vi "RealSense_HelloWorld_Left_Right_unrectified.vi"() -> ()   [LabVIEW 2017]
doc: "This demo shows how to connect a RealSense D4xx Stereo Depth Camera, and stream the LEFT and the RIGHT raw unrectified images."
uses:
  <vilib>/picture/picture.llb/Draw True-Color Pixmap.vi
  libRealSense3.lvlib
panel:
  in  "autoexposure":bool
  in  "Gain (16-248)":sgl=16.0
  in  "Exposure,us":sgl=33000.0
  in  "Tab Control":enum32{"Monochrome L+R", "Intensity Chart L"}(tab)
  in  "Zoom Factor":sgl=0.29
  out "Unrect L":picture
  out "Unrect R":picture
  out "LEFT IMAGE":sgl[][](graph)
  out "RIGHT IMAGE":sgl[][](graph)
  out "iteration":i32=1
  in  "stop":bool=TRUE
  out "release frame error":string="No Error"
  out "Capture1 Error":string="No Error"
  out "Config error":string="No Error\rNo Error"
  out "init results":T1={"camera name"="Intel RealSense 415", "camera S/N"="725112060291", "F/W"="05.08.09.00", "Sensor name"="Stereo Module", "api_version"=20710, "rscontext"=657762304, "device_list"=395444960, "device count"=2, "Dev out"=657678208, "sensor_list"=657686400, "sensor count"=2, "Sensor out"=657915824}
  out "init error":string="No Error\rNo Error\rNo Error\rNo Error\rNo Error\rNo Error\rNo Error\rNo Error\rNo Error\rNo Error\rNo Error"
  out "Close Error":string="No Error\rNo Error\rNo Error\rNo Error"
  out "Start Error":string="No Error\rNo Error\rNo Error"
  out "Capture2 error":string="No Error"
  in  "Select Resolution":u16(ring)=3 items=["960 x 540 @15fps", "960 x 540 @25fps", "1920 x 1080 @15fps", "1920 x 1080 @25fps"]
  # "RealSense Hello World: Left-Right UnRectified"
  # "This demo shows how to connect a RealSense D4xx Stereo Depth Camera, and stream the LEFT and the RIGHT raw unrectified images. Zoom in and scroll the horizontal/vertical bar to look at different parts of image. The images are the input images to the stereo algorithm. They are not rectified by ASIC.  They can be used to look at raw image quality before any processing."
  # "Use this to ZOOM and move image"
  # "Use this to ZOOM and move image"
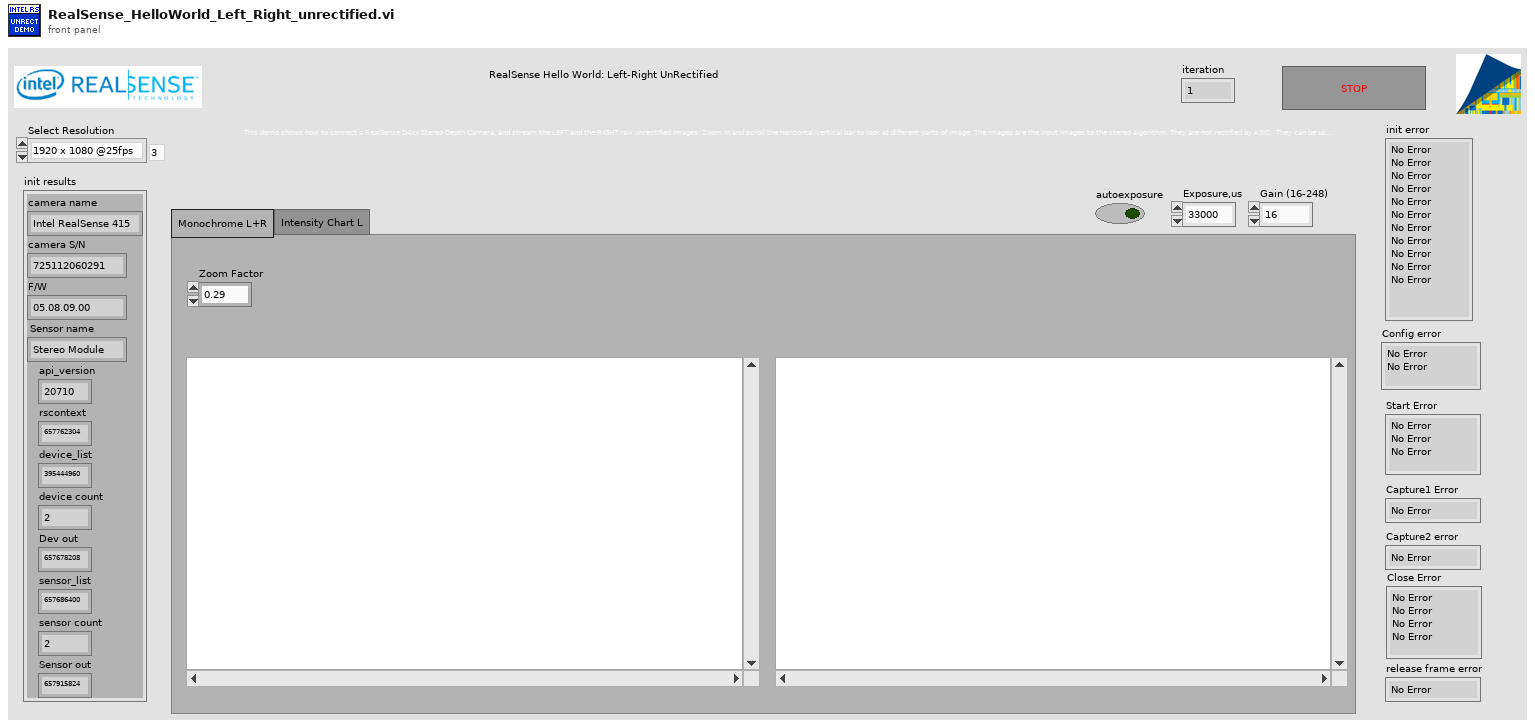
[diagram p1: front panel]
types:
  T1 = cluster{"camera name":string, "camera S/N":string, "F/W":string, "Sensor name":string, "api_version":i32, "rscontext":u64, "device_list":u64, "device count":i32, "Dev out":u64, "sensor_list":u64, "sensor count":i32, "Sensor out":u64}
  T2 = enum16{"Depth", "Color (ext.)", "Color (left) ", "IR Left", "IR Right", "IR Left (Y16)", "IR Right (Y16)"}
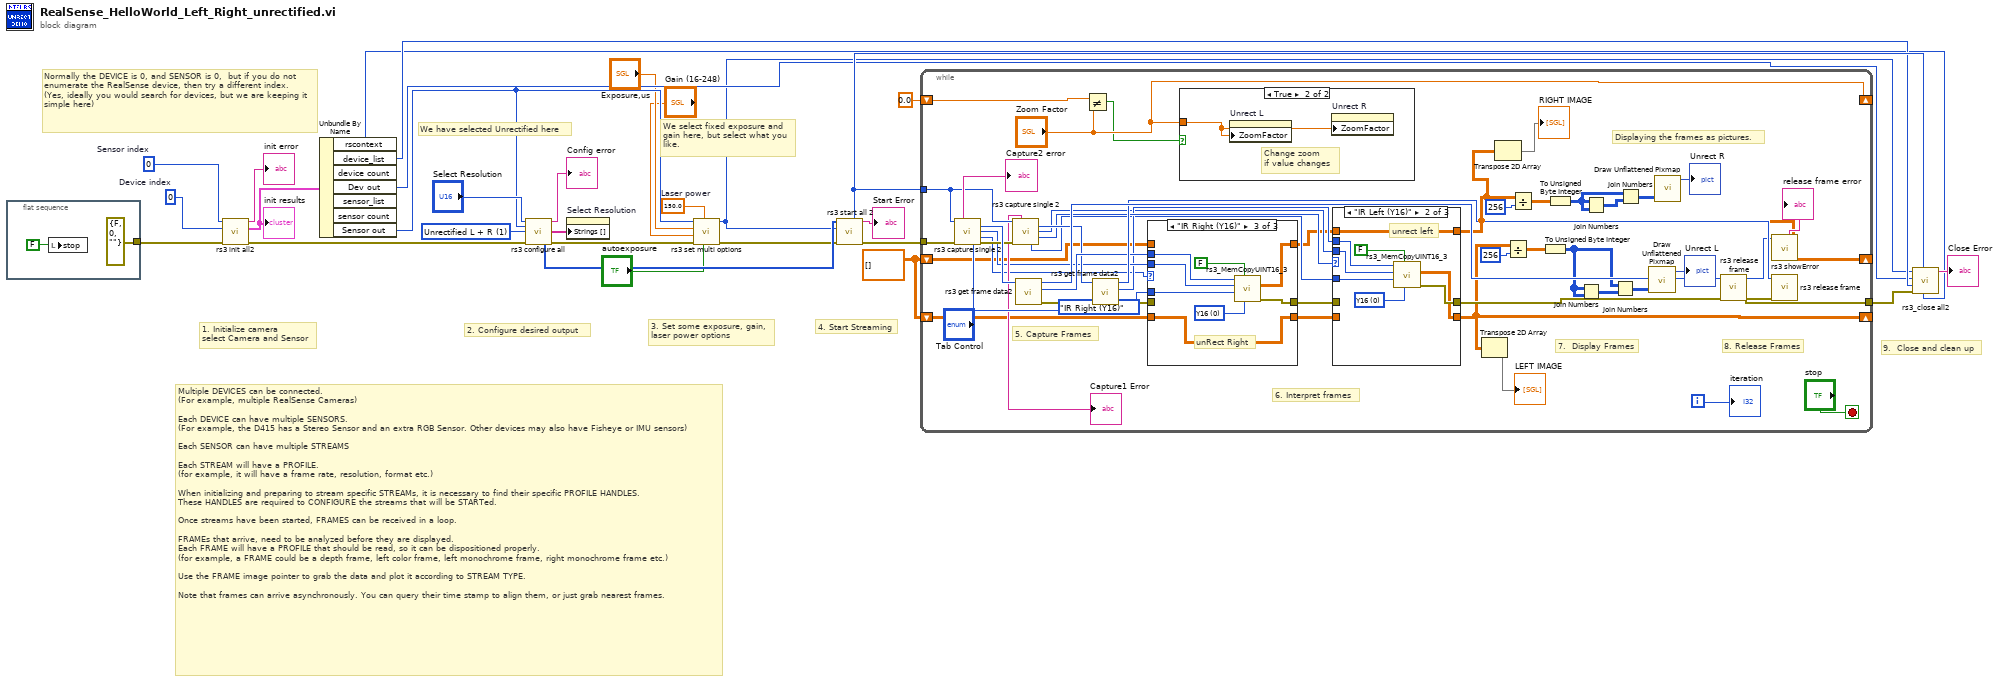
[diagram p0: block diagram]
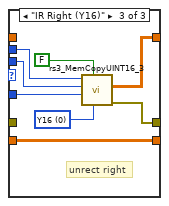
[diagram p4: hidden frame]
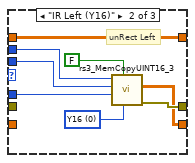
[diagram p6: hidden frame]
diagram:
  w29 = 0  # Device index
  w28 = 0  # Sensor index
  w4 = sgl 150.0  # Laser power
  w10 = u16 1 items=["Depth + Left Color", "Unrectified L + R", "Rectified L + R"] ("Stream selection")
  w11 = sgl[][] [] ("2D Array Output")
  # "We select fixed exposure and gain here, but select what you like."
  # "We have selected Unrectified here"
  # "Normally the DEVICE is 0, and SENSOR is 0,  but if you do not enumerate the RealSense device, then try a different index.\n(Yes, ideally you would search for devices, but we are keeping it simple here)"
  # "Multiple DEVICES can be connected. \n(For example, multiple RealSense Cameras)\n\nEach DEVICE can have multiple SENSORS. \n(For example, the D415 has a Stereo Sensor and an extra RGB Sensor. Other devices may also have Fisheye or IMU sensors) \n\nEach SENSOR can have multiple STREAMS\n\nEach STREAM will have a PROFILE. \n(for example, it will have a frame rate, resolution, format etc.)\n\nWhen initializing and preparing to stream specific STREAMs, it is necessary to find their specific PROFILE HANDLES.\nThese HANDLES are required to CONFIGURE the streams that will be STARTed. \n\nOnce streams have been started, FRAMES can be received in a loop. \n \nFRAMEs that arrive, need to be analyzed before they are displayed. \nEach FRAME will have a PROFILE that should be read, so it can be dispositioned properly.\n(for example, a FRAME could be a depth frame, left color frame, left monochrome frame, right monochrome frame etc.)\n\nUse the FRAME image pointer to grab the data and plot it according to STREAM TYPE.\n\nNote that frames can arrive asynchronously. You can query their time stamp to align them, or just grab nearest frames."
  # "9.  Close and clean up"
  # "4. Start Streaming"
  # "3. Set some exposure, gain, \nlaser power options"
  # "2. Configure desired output"
  # "1. Initialize camera\nselect Camera and Sensor"
  n1 = flat-sequence {
    tunnel: [errorcluster {"status"=FALSE, "code"=0, "source"=""} ("error in")] -> w12
    frame #0 {
      n2 = local write "stop"(FALSE ("stop")) -> ()
    }
  }
  n3 = call "rs3 init all2.vi"("error in"=w12, "Select Device"=w29, "Select Sensor"=w28) -> ("error out"=w27:errorcluster, "init results"=w20:T1, "init error"=→"init error":string)  [unwired: 2 in, 4 out]
  "init results" <- w20
  n4 = Unbundle By Name(w20) -> ("rscontext"=w18:u64, "device_list"=w19:u64, "Dev out"=w15:u64, "Sensor out"=w7:u64)  [unwired: 3 out]
  n5 = call "rs3 configure all.vi"("Select Resolution"="Select Resolution", "Sensor in"=w7, "Stream selection"=w10, "error in (no error)"=w27) -> ("config error"=→"Config error":string, "Output stream"=w13:string[], "Stream Profile Handles"=w26:u64[], "error out"=w9:errorcluster)  [unwired: 2 in, 6 out]
  n6 = property on="Select Resolution" class="Ring (strict)"("Strings []"=w13) -> ()  [unwired: 2 in, 2 out]
  n7 = call "rs3 set multi options.vi"("autoexposure"="autoexposure", "Laser power, mW (0-360)"=w4, "error in (no error)"=w9, "Gain(16-248)"="Gain (16-248)", "Exposure, us"="Exposure,us", "Sensor in"=w7) -> ("error out"=w8:errorcluster, "Sensor out"=w6:u64)  [unwired: 3 in, 1 out]
  n8 = call "rs3 start all 2.vi"("error in (no error)"=w8, "Sensor in"=w6, "Stream profile array"=w26) -> ("error out"=w14:errorcluster, "Config Error"=→"Start Error":string, "queue out"=w25:u64)  [unwired: 5 in, 1 out]
  n9 = while {
    tunnel: w25 -> [w68]
    tunnel: w14 -> [w81]
    tunnel: [w73] -> w24
    shift-right: [w33] -> _
    shift-left: w11 -> [w54]
    shift-right: [w35] -> _
    shift-left: w11 -> [w52]
    shift-right: ["Zoom Factor"] -> _
    shift-left: sgl 0.0 ("Zoom Factor") -> [w38]
    i -> [w79]
    stop <- "stop" stop-if-true
    (unwired) T2."IR Right (Y16)" ("Stream type")
    # "Displaying the frames as pictures."
    # "8. Release Frames"
    # "7.  Display Frames"
    # "6. Interpret frames"
    # "5. Capture Frames"
    n10 = call "rs3 capture single 2.vi"("queue in"=w68, "error in (no error)"=w81) -> ("Capture Error"=→"Capture2 error":string, "frame out"=w78:u64, "width"=w65:i32, "Stream type"=w55:T2, "height"=w75:i32, "error out"=w69:errorcluster)  [unwired: 2 in, 6 out]
    n11 = call "rs3 capture single 2.vi"("queue in"=w68, "error in (no error)"=w69) -> ("Capture Error"=→"Capture1 Error":string, "frame out"=w66:u64, "width"=w57:i32, "Stream type"=w59:T2, "height"=w56:i32)  [unwired: 2 in, 7 out]
    n12 = call "rs3 get frame data2.vi"("frame in"=w78) -> ("error out"=w72:errorcluster, "image pointer out"=w76:u64, "Frame out"=w80:u64)  [unwired: 7 in, 1 out]
    n13 = Not Equal?(x=w38, y="Zoom Factor") -> (x != y?=w36:bool)
    n14 = call "rs3 get frame data2.vi"("error in (no error)"=w72, "frame in"=w66) -> ("error out"=w71:errorcluster, "image pointer out"=w58:u64, "Frame out"=w77:u64)  [unwired: 6 in, 1 out]
    n15 = case shown="\"IR Right (Y16)\"" w55 {
      tunnel: [w104 w111 w119] -> w61
      tunnel: w76 -> [_ w110 w118]
      tunnel: w65 -> [_ w109 w117]
      tunnel: w75 -> [_ w108 w116]
      tunnel: w71 -> [w104 _ _]
      tunnel: [w103 w107 w114] -> w53
      tunnel: w54 -> [w103 _ w114]
      tunnel: w52 -> [w102 w106 _]
      tunnel: [w102 w106 w115] -> w51
      frame "Color (ext.)", Default {
      }
      frame "IR Left (Y16)" {
        w112 = u16 0 items=["Y16", "Y8"] ("Image format")
        # "unRect Left"
        n16 = call "rs3_MemCopyUINT16_3.vi"("Image format"=w112, "Transpose"=FALSE, "Depth Y"=w108, "Depth X"=w109, "Zimage pointer"=w110) -> ("error out"=w111:errorcluster, "2D Array Output"=w107:sgl[][])  [unwired: 3 in, 2 out]
      }
      frame "IR Right (Y16)" {
        w120 = u16 0 items=["Y16", "Y8"] ("Image format")
        # "unRect Right"
        n17 = call "rs3_MemCopyUINT16_3.vi"("Image format"=w120, "Transpose"=FALSE, "Depth Y"=w116, "Depth X"=w117, "Zimage pointer"=w118) -> ("error out"=w119:errorcluster, "2D Array Output"=w115:sgl[][])  [unwired: 3 in, 2 out]
      }
    }
    n18 = case shown="True" w36 {
      tunnel: "Zoom Factor" -> [_ w82]
      frame False {
      }
      frame True {
        # "Change zoom\nif value changes"
        n19 = property on="Unrect L" class="Pict"("ZoomFactor"=w82) -> ()  [unwired: 2 in, 2 out]
        n20 = property on="Unrect R" class="Pict"("ZoomFactor"=w82) -> ()  [unwired: 2 in, 2 out]
      }
    }
    n21 = case shown="\"IR Left (Y16)\"" w59 {
      tunnel: [w85 w92 w100] -> w60
      tunnel: w58 -> [_ w91 w99]
      tunnel: w57 -> [_ w90 w98]
      tunnel: w56 -> [_ w89 w97]
      tunnel: w61 -> [w85 _ _]
      tunnel: w53 -> [w84 _ w95]
      tunnel: [w84 w88 w95] -> w33
      tunnel: [w83 w87 w96] -> w35
      tunnel: w51 -> [w83 w87 _]
      frame "Color (ext.)", Default {
      }
      frame "IR Left (Y16)" {
        w93 = u16 0 items=["Y16", "Y8"] ("Image format")
        # "unrect left"
        n22 = call "rs3_MemCopyUINT16_3.vi"("Image format"=w93, "Transpose"=FALSE, "Depth Y"=w89, "Depth X"=w90, "Zimage pointer"=w91) -> ("error out"=w92:errorcluster, "2D Array Output"=w88:sgl[][])  [unwired: 3 in, 2 out]
      }
      frame "IR Right (Y16)" {
        w101 = u16 0 items=["Y16", "Y8"] ("Image format")
        # "unrect right"
        n23 = call "rs3_MemCopyUINT16_3.vi"("Image format"=w101, "Transpose"=FALSE, "Depth Y"=w97, "Depth X"=w98, "Zimage pointer"=w99) -> ("error out"=w100:errorcluster, "2D Array Output"=w96:sgl[][])  [unwired: 3 in, 2 out]
      }
    }
    n24 = Transpose 2D Array(2D array=w33) -> (transposed array=→"LEFT IMAGE":sgl[][])
    n25 = Transpose 2D Array(2D array=w35) -> (transposed array=→"RIGHT IMAGE":sgl[][])
    n26 = Divide(x=w33, y=256) -> (x/y=w50:sgl[][])
    n27 = Divide(x=w35, y=256) -> (x/y=w43:sgl[][])
    n28 = To Unsigned Byte Integer(number=w50) -> (unsigned 8bit integer=w47:u8[][])
    n29 = To Unsigned Byte Integer(number=w43) -> (unsigned 8bit integer=w45:u8[][])
    n30 = Join Numbers(hi=w47, lo=w47) -> ((hi.lo)=w48:u16[][])
    n31 = Join Numbers(hi=w45, lo=w45) -> ((hi.lo)=w42:u16[][])
    n32 = Join Numbers(hi=w47, lo=w48) -> ((hi.lo)=w40:u32[][])
    n33 = Join Numbers(hi=w45, lo=w42) -> ((hi.lo)=w39:u32[][])
    n34 = call-poly <vilib>:"Draw Unflattened Pixmap.vi"("data (RGB format)"=w40) -> ("new picture"=→"Unrect L":picture)  [unwired: 8 in]
    n35 = call-poly <vilib>:"Draw Unflattened Pixmap.vi"("data (RGB format)"=w39) -> ("new picture"=→"Unrect R":picture)  [unwired: 8 in]
    n36 = call "rs3 release frame.vi"("error in (no error)"=w60, "Frame"=w80) -> ("error out"=w74:errorcluster, "error"=w64:u64)  [unwired: 8 in]
    n37 = call "rs3 showError.vi"("error"=w64) -> ("Error summary"=→"release frame error":string)  [unwired: 6 in, 4 out]
    n38 = call "rs3 release frame.vi"("error in (no error)"=w74, "Frame"=w77) -> ("error out"=w73:errorcluster)  [unwired: 8 in, 1 out]
    "iteration" <- w79
  }
  n39 = call "rs3_close all2.vi"("rscontext"=w18, "queue in"=w25, "error in (no error)"=w24, "device_list"=w19, "Dev in"=w15, "Sensor in"=w6) -> ("Close Error"=→"Close Error":string)  [unwired: 4 in, 1 out]
